vi "custom.vi"() -> ()   [LabVIEW 2009]
panel:
  out "Turning Turret":bool
  in  "Exit":bool
  in  "Abort\n Scan":bool
  out "Scanning":bool
  out "error out":errorcluster
  out "Status":string
  out "Emulating":bool
  out "Initialized":bool
  in  "Force\nInitialization":bool
  in  "Initialize":bool
  out "Current UniqueID":string
  in  "Mono ID":string(combo)
  in  "Switch \nTurret":bool
  out "Wavelength (nm)":dbl
  out "Grating Index":i32
  in  "Select Grating Blaze":string(combo)
  out "Current Blaze":string caption="Grating Blaze"
  out "Grating Density":dbl
  in  "Time Per Step":dbl=1.0 min=1.0 max=5000.0 step=1.0
  in  "Wavelength\n   Step Size":dbl=1.0 min=0.1 max=100.0
  in  "Ending\nWavelength":dbl=500.0 min=201.0 max=3000.0
  in  "Starting\nWavelength":dbl=450.0 min=18.0 max=2500.0
  in  "Target\nWavelength":dbl=450.0 min=18.0 max=3000.0
  in  "Increment":dbl=10.0 min=0.1 max=50.0
  out "Incrementing Down":bool
  out "Incrementing Up":bool
  out "Changing Wavelength":bool
  in  "Scan":bool
  in  "Increment Down":bool
  in  "Increment Up":bool
  in  "Change Wavelength":bool
  out "Drive Control Engaged":bool
  in  "Change \nGrating":bool
  in  "Enable\nDrive":bool
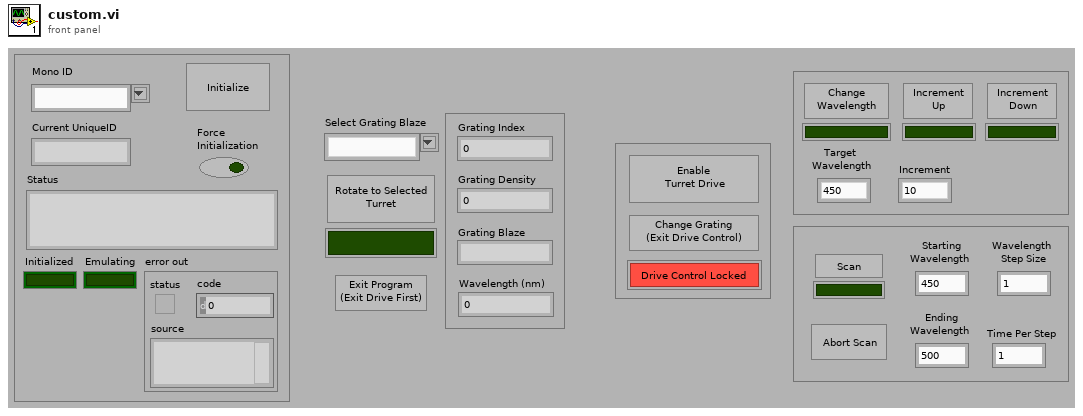
[diagram p1: front panel]
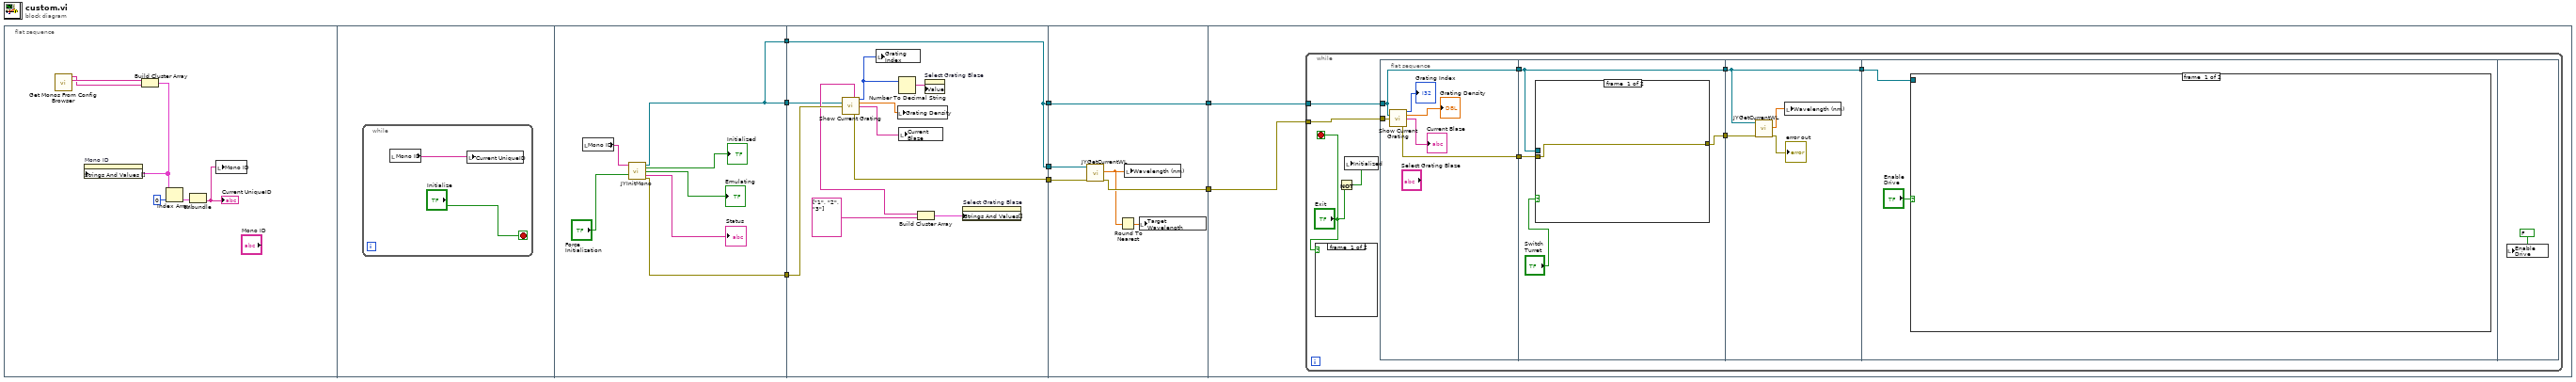
[diagram p0: block diagram]
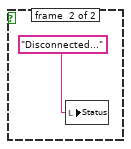
[diagram p2: hidden frame]
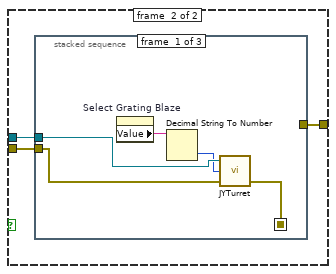
[diagram p3: hidden frame]
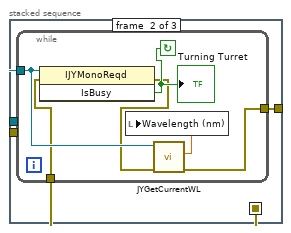
[diagram p4: hidden frame]
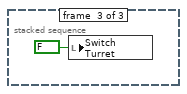
[diagram p5: hidden frame]
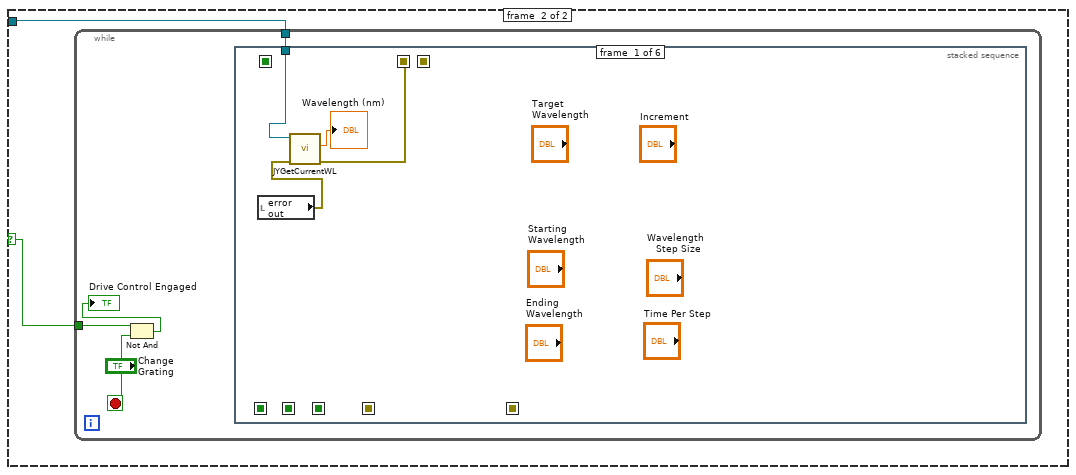
[diagram p6: hidden frame]
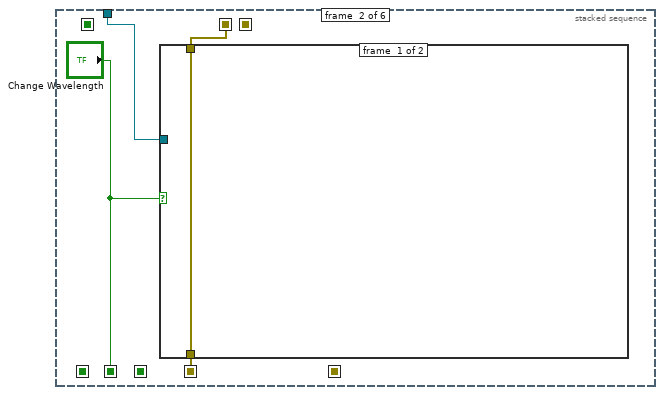
[diagram p7: hidden frame]
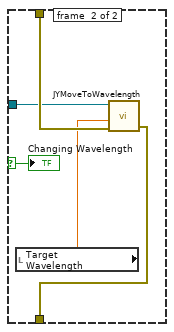
[diagram p8: hidden frame]
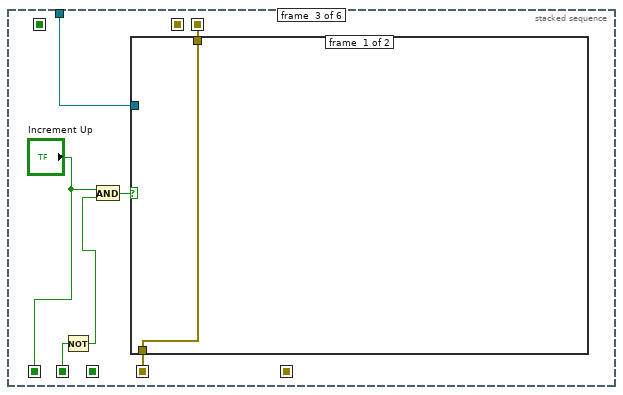
[diagram p9: hidden frame]
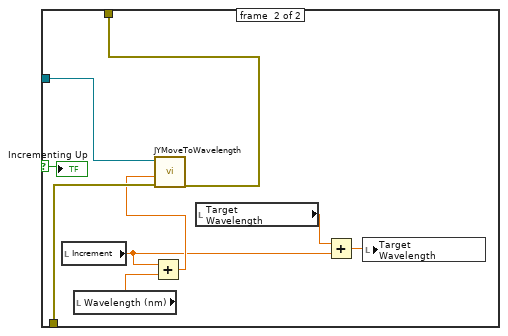
[diagram p10: hidden frame]
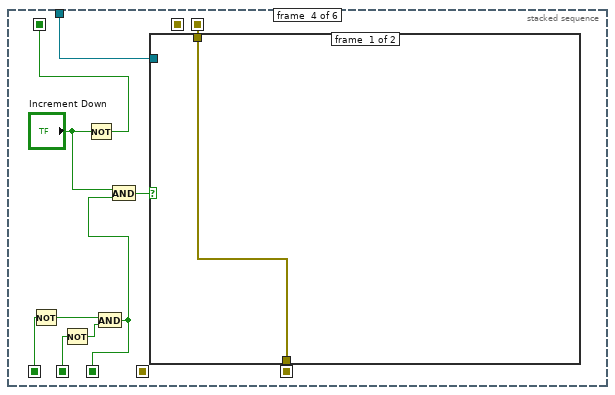
[diagram p11: hidden frame]
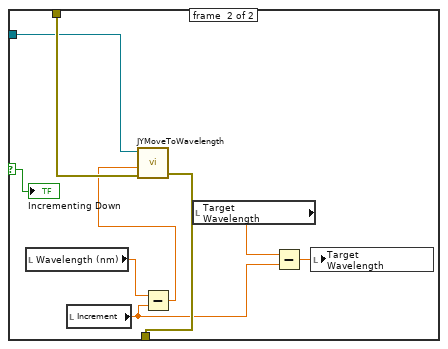
[diagram p12: hidden frame]
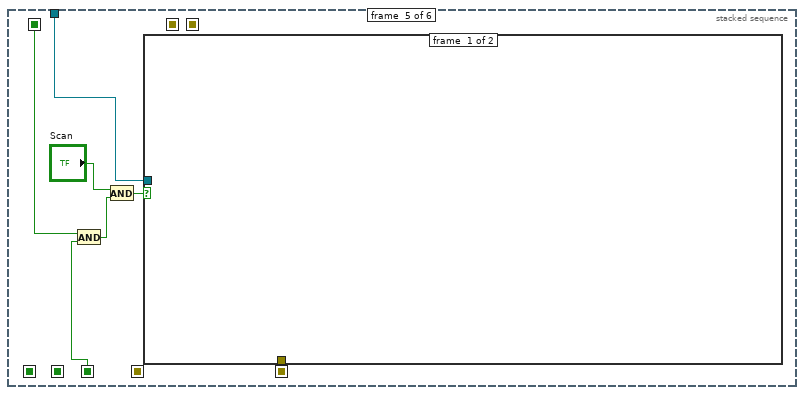
[diagram p13: hidden frame]
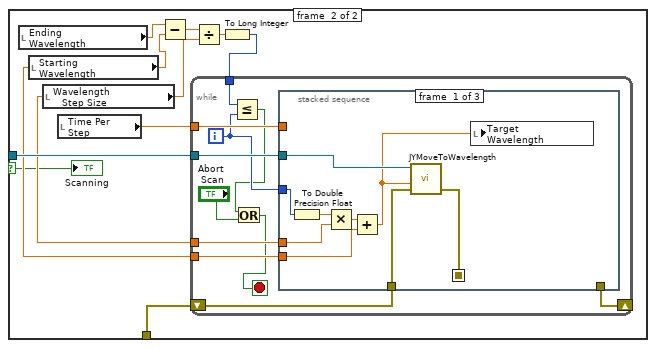
[diagram p14: hidden frame]
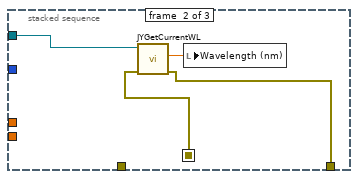
[diagram p15: hidden frame]
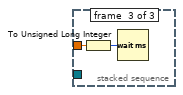
[diagram p16: hidden frame]
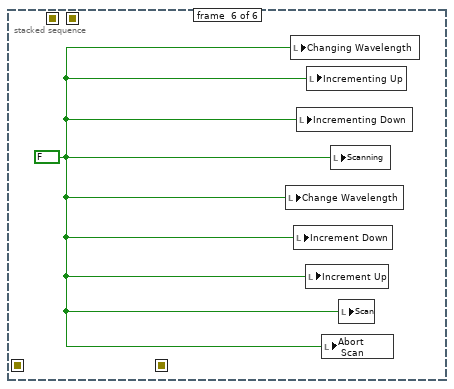
[diagram p17: hidden frame]
diagram:
  n1 = flat-sequence {
    tunnel: [w18] -> w8
    tunnel: [w17] -> w7
    tunnel: [w17] -> w2
    tunnel: w8 -> [w34]
    tunnel: w7 -> [w25]
    tunnel: [w32] -> w4
    tunnel: [w24] -> w6
    tunnel: w2 -> [w24]
    tunnel: [w24] -> w1
    tunnel: w6 -> [w40]
    tunnel: [w37] -> w5
    tunnel: w4 -> [w39]
    tunnel: [w38] -> w3
    tunnel: w1 -> [w37]
    tunnel: w5 -> [w41]
    tunnel: w3 -> [w42]
    frame #0 {
      n2 = call "Get Monos From Config Browser.vi"() -> ("UniqueIDs"=w13:string[], "Mono ID"=w14:string[])  [unwired: 3 in, 1 out]
      n3 = Build Cluster Array(w14, w13) -> (w11:cluster{"String":string, "String":string}[])
      n4 = property on="Mono ID" class="CmbBox"("Strings And Values []"=w11) -> ()  [unwired: 2 in, 2 out]
      n5 = Index Array(array=w11, index=0) -> (element=w12:cluster{"String":string, "String":string})
      n6 = Unbundle(w12) -> ("String"=w9:string)  [unwired: 1 out]
      "Current UniqueID" <- w9
      n7 = local write "Mono ID"(w9) -> ()
    }
    frame #1 {
      n8 = while {
        stop <- "Initialize" stop-if-true
        n9 = local read "Mono ID"() -> (w16:string)
        n10 = local write "Current UniqueID"(w16) -> ()
      }
    }
    frame #2 {
      n11 = local read "Mono ID"() -> (w22:string)
      n12 = call "JYInitMono.vi"("Unique ID"=w22, "Force Init"="Force\nInitialization") -> ("Mono RefNum out"=w17:refnum<k7>, "Initialized"=→"Initialized":bool, "Emulating"=→"Emulating":bool, "Status"=→"Status":string, "error out"=w18:errorcluster)  [unwired: 9 in]
    }
    frame #3 {
      n13 = call "Show Current Grating.vi"("Refnum in"=w25, "error in (no error)"=w34) -> ("Blazes"=w29:string[], "Grating Index"=w28:i32, "Current Grating"=w27:dbl, "Current Blaze"=w26:string, "error out"=w32:errorcluster)  [unwired: 5 in, 4 out]
      n14 = local write "Grating Index"(w28) -> ()
      n15 = local write "Grating Density"(w27) -> ()
      n16 = Number To Decimal String(number=w28) -> (decimal integer string=w31:string)  [unwired: 1 in]
      n17 = local write "Current Blaze"(w26) -> ()
      n18 = Build Cluster Array(w29, string[] ["1", "2", "3"]) -> (w30:cluster{"String":string, string}[])
      n19 = property on="Select Grating Blaze" class="CmbBox"("Value"=w31) -> ()  [unwired: 2 in, 2 out]
      n20 = property on="Select Grating Blaze" class="CmbBox"("Strings And Values[]"=w30) -> ()  [unwired: 2 in, 2 out]
    }
    frame #4 {
      n21 = call "JYGetCurrentWL.vi"("error in (no error)"=w39, "JYMONOLib.IJYMonoReqd"=w40) -> ("error out"=w38:errorcluster, "Current WL"=w36:dbl)  [unwired: 6 in, 2 out]
      n22 = Round To Nearest(number=w36) -> (nearest integer value=w35:dbl)
      n23 = local write "Wavelength (nm)"(w36) -> ()
      n24 = local write "Target\nWavelength"(w35) -> ()
    }
    frame #5 {
      n25 = while {
        tunnel: w41 -> [w51]
        tunnel: w42 -> [w50]
        stop <- "Exit" stop-if-true
        n26 = case shown="False" "Exit" {
          frame #0 {
          }
          frame #1 {
            n27 = local write "Status"("Disconnected...") -> ()
          }
        }
        n28 = Not(x="Exit") -> (.not. x?=w44:bool)
        n29 = local write "Initialized"(w44) -> ()
        n30 = flat-sequence {
          tunnel: w51 -> [w53]
          tunnel: w50 -> [w55]
          tunnel: [w54] -> w49
          tunnel: [w53] -> w47
          tunnel: w49 -> [w62]
          tunnel: [w60] -> w48
          tunnel: w47 -> [w61]
          tunnel: [w61] -> w46
          tunnel: w48 -> [w85]
          tunnel: w46 -> [w84]
          tunnel: [w84] -> w45
          tunnel: w45 -> [w87]
          frame #0 {
            n31 = call "Show Current Grating.vi"("Refnum in"=w53, "error in (no error)"=w55) -> ("Grating Index"=→"Grating Index":i32, "Current Grating"=→"Grating Density":dbl, "Current Blaze"=→"Current Blaze":string, "error out"=w54:errorcluster)  [unwired: 5 in, 5 out]
          }
          frame #1 {
            n32 = case shown="True" "Switch \nTurret" {
              tunnel: w62 -> [w63 w66]
              tunnel: w61 -> [_ w65]
              tunnel: [w63 w64] -> w60
              frame #0 {
              }
              frame #1 {
                n33 = stacked-sequence {
                  seq-local: [w69 _ _] -> [_ w73 _]
                  tunnel: w66 -> [w71 _ _]
                  tunnel: w65 -> [w70 w74 _]
                  tunnel: [_ w72 _] -> w64
                  frame #0 {
                    n34 = property on="Select Grating Blaze" class="CmbBox"() -> ("Value"=w68:string)  [unwired: 2 in, 2 out]
                    n35 = Decimal String To Number(string=w68) -> (number=w67:i32)  [unwired: 2 in, 1 out]
                    n36 = call "JYTurret.vi"("error in (no error)"=w71, "Grating Index"=w67, "RefNum In"=w70) -> ("error out"=w69:errorcluster)  [unwired: 2 out]
                  }
                  frame #1 {
                    n37 = while {
                      tunnel: w74 -> [w80]
                      tunnel: w73 -> [w78]
                      tunnel: [w75] -> w72
                      stop <- w77 continue-if-true
                      n38 = invoke class="IJYMonoReqd" method="IsBusy"(reference=w80, error in=w78) -> (error out=w76:errorcluster, "IsBusy"=w77:bool)  [unwired: 1 in, 1 out]
                      "Turning Turret" <- w77
                      n39 = call "JYGetCurrentWL.vi"("error in (no error)"=w76, "JYMONOLib.IJYMonoReqd"=w80) -> ("error out"=w75:errorcluster, "Current WL"=w79:dbl)  [unwired: 6 in, 2 out]
                      n40 = local write "Wavelength (nm)"(w79) -> ()
                    }
                  }
                  frame #2 {
                    n41 = local write "Switch \nTurret"(FALSE ("Switch \nTurret")) -> ()
                  }
                }
              }
            }
          }
          frame #2 {
            n42 = call "JYGetCurrentWL.vi"("error in (no error)"=w85, "JYMONOLib.IJYMonoReqd"=w84) -> ("error out"=→"error out":errorcluster, "Current WL"=w82:dbl)  [unwired: 6 in, 2 out]
            n43 = local write "Wavelength (nm)"(w82) -> ()
          }
          frame #3 {
            n44 = case shown="False" "Enable\nDrive" {
              selector: "Enable\nDrive" -> [_ w89]
              tunnel: w87 -> [_ w88]
              frame #0 {
              }
              frame #1 {
                n45 = while {
                  tunnel: w89 -> [w91]
                  tunnel: w88 -> [w90]
                  stop <- "Change \nGrating" stop-if-true
                  n46 = Not And(1:"Change \nGrating", 2:w91) -> (0:→"Drive Control Engaged":bool)
                  n47 = stacked-sequence {
                    seq-local: [_ "Change Wavelength" _ _ _ _] -> [_ _ w114 w135 _ _]
                    seq-local: [_ _ "Increment Up" _ _ _] -> [_ _ _ w134 _ _]
                    seq-local: [_ _ _ w129 _ _] -> [_ _ _ _ w152 _]
                    seq-local: [_ _ _ w128 _ _] -> [_ _ _ _ w151 _]
                    seq-local: [w95 _ _ _ _ _] -> [_ w100 _ _ _ _]
                    seq-local: [_ w98 _ _ _ _] -> [_ _ w110 _ _ _]
                    seq-local: [_ _ w108 _ _ _] -> [_ _ _ w127 _ _]
                    seq-local: [_ _ _ w125 _ _] -> [_ _ _ _ w147 _]
                    tunnel: w90 -> [w94 w99 w109 w126 w146 _]
                    frame #0 {
                      n48 = local read "error out"() -> (w97:errorcluster)
                      n49 = call "JYGetCurrentWL.vi"("error in (no error)"=w97, "JYMONOLib.IJYMonoReqd"=w94) -> ("error out"=w95:errorcluster, "Current WL"=→"Wavelength (nm)":dbl)  [unwired: 6 in, 2 out]
                    }
                    frame #1 {
                      n50 = case shown="True" "Change Wavelength" {
                        selector: "Change Wavelength" -> [_ w103]
                        tunnel: w100 -> [w102 w107]
                        tunnel: w99 -> [_ w106]
                        tunnel: [w102 w105] -> w98
                        frame #0 {
                        }
                        frame #1 {
                          n51 = local read "Target\nWavelength"() -> (w104:dbl)
                          n52 = call "JYMoveToWavelength.vi"("error in (no error)"=w107, "Target WL"=w104, "RefNum In"=w106) -> ("error out"=w105:errorcluster)  [unwired: 1 in, 2 out]
                          "Changing Wavelength" <- w103
                        }
                      }
                    }
                    frame #2 {
                      n53 = Not(x=w114) -> (.not. x?=w111:bool)
                      n54 = And(x="Increment Up", y=w111) -> (x .and. y?=w113:bool)
                      n55 = case shown="True" w113 {
                        selector: w113 -> [_ w116]
                        tunnel: w110 -> [w115 w124]
                        tunnel: w109 -> [_ w122]
                        tunnel: [w115 w121] -> w108
                        frame #0 {
                        }
                        frame #1 {
                          n56 = local read "Increment"() -> (w119:dbl)
                          n57 = local read "Wavelength (nm)"() -> (w120:dbl)
                          n58 = Add(x=w119, y=w120) -> (x+y=w123:dbl)
                          n59 = call "JYMoveToWavelength.vi"("error in (no error)"=w124, "Target WL"=w123, "RefNum In"=w122) -> ("error out"=w121:errorcluster)  [unwired: 1 in, 2 out]
                          n60 = local read "Target\nWavelength"() -> (w118:dbl)
                          n61 = Add(x=w118, y=w119) -> (x+y=w117:dbl)
                          n62 = local write "Target\nWavelength"(w117) -> ()
                          "Incrementing Up" <- w116
                        }
                      }
                    }
                    frame #3 {
                      n63 = Not(x=w134) -> (.not. x?=w132:bool)
                      n64 = Not(x=w135) -> (.not. x?=w133:bool)
                      n65 = Not(x="Increment Down") -> (.not. x?=w129:bool)
                      n66 = And(x=w132, y=w133) -> (x .and. y?=w128:bool)
                      n67 = And(x="Increment Down", y=w128) -> (x .and. y?=w131:bool)
                      n68 = case shown="True" w131 {
                        selector: w131 -> [_ w137]
                        tunnel: w127 -> [w136 w145]
                        tunnel: w126 -> [_ w143]
                        tunnel: [w136 w142] -> w125
                        frame #0 {
                        }
                        frame #1 {
                          n69 = local read "Wavelength (nm)"() -> (w141:dbl)
                          n70 = local read "Increment"() -> (w139:dbl)
                          n71 = Subtract(x=w141, y=w139) -> (x-y=w144:dbl)
                          n72 = call "JYMoveToWavelength.vi"("error in (no error)"=w145, "Target WL"=w144, "RefNum In"=w143) -> ("error out"=w142:errorcluster)  [unwired: 1 in, 2 out]
                          n73 = local read "Target\nWavelength"() -> (w140:dbl)
                          n74 = Subtract(x=w140, y=w139) -> (x-y=w138:dbl)
                          n75 = local write "Target\nWavelength"(w138) -> ()
                          "Incrementing Down" <- w137
                        }
                      }
                    }
                    frame #4 {
                      n76 = And(x=w152, y=w151) -> (x .and. y?=w149:bool)
                      n77 = And(x="Scan", y=w149) -> (x .and. y?=w150:bool)
                      n78 = case shown="True" w150 {
                        selector: w150 -> [_ w153]
                        tunnel: w147 -> [_ w158]
                        tunnel: w146 -> [_ w157]
                        frame #0 {
                        }
                        frame #1 {
                          n79 = local read "Ending\nWavelength"() -> (w160:dbl)
                          n80 = local read "Starting\nWavelength"() -> (w155:dbl)
                          n81 = local read "Wavelength\n   Step Size"() -> (w156:dbl)
                          n82 = local read "Time Per Step"() -> (w159:dbl)
                          n83 = Subtract(x=w160, y=w155) -> (x-y=w162:dbl)
                          n84 = Divide(x=w162, y=w156) -> (x/y=w161:dbl)
                          n85 = To Long Integer(number=w161) -> (32bit integer=w154:i32)
                          n86 = while {
                            tunnel: w155 -> [w169]
                            tunnel: w159 -> [w173]
                            shift-right: [w168] -> _
                            shift-left: w158 -> [w172]
                            tunnel: w157 -> [w171]
                            tunnel: w156 -> [w170]
                            tunnel: w154 -> [w164]
                            i -> [w167]
                            stop <- w165 stop-if-true
                            n87 = Less Or Equal?(x=w164, y=w167) -> (x <= y?=w166:bool)
                            n88 = Or(x=w166, y="Abort\n Scan") -> (x .or. y?=w165:bool)
                            n89 = stacked-sequence {
                              seq-local: [w175 _ _] -> [_ w184 _]
                              tunnel: w173 -> [_ _ w187]
                              tunnel: w172 -> [w182 _ _]
                              tunnel: w171 -> [w181 w185 _]
                              tunnel: w170 -> [w180 _ _]
                              tunnel: w167 -> [w179 _ _]
                              tunnel: w169 -> [w176 _ _]
                              tunnel: [_ w183 _] -> w168
                              frame #0 {
                                n90 = To Double Precision Float(number=w179) -> (double precision float=w178:dbl)
                                n91 = Multiply(x=w178, y=w180) -> (x*y=w177:dbl)
                                n92 = Add(x=w177, y=w176) -> (x+y=w174:dbl)
                                n93 = call "JYMoveToWavelength.vi"("error in (no error)"=w182, "Target WL"=w174, "RefNum In"=w181) -> ("error out"=w175:errorcluster)  [unwired: 1 in, 2 out]
                                n94 = local write "Target\nWavelength"(w174) -> ()
                              }
                              frame #1 {
                                n95 = call "JYGetCurrentWL.vi"("error in (no error)"=w184, "JYMONOLib.IJYMonoReqd"=w185) -> ("error out"=w183:errorcluster, "Current WL"=w186:dbl)  [unwired: 6 in, 2 out]
                                n96 = local write "Wavelength (nm)"(w186) -> ()
                              }
                              frame #2 {
                                n97 = To Unsigned Long Integer(number=w187) -> (unsigned 32bit integer=w188:u32)
                                n98 = Wait (ms)(milliseconds to wait=w188) -> ()  [unwired: 1 out]
                              }
                            }
                          }
                          "Scanning" <- w153
                        }
                      }
                    }
                    frame #5 {
                      w189 = FALSE
                      n99 = local write "Change Wavelength"(w189) -> ()
                      n100 = local write "Changing Wavelength"(w189) -> ()
                      n101 = local write "Increment Down"(w189) -> ()
                      n102 = local write "Incrementing Down"(w189) -> ()
                      n103 = local write "Increment Up"(w189) -> ()
                      n104 = local write "Incrementing Up"(w189) -> ()
                      n105 = local write "Abort\n Scan"(w189) -> ()
                      n106 = local write "Scanning"(w189) -> ()
                      n107 = local write "Scan"(w189) -> ()
                    }
                  }
                }
              }
            }
          }
          frame #4 {
            n108 = local write "Enable\nDrive"(FALSE) -> ()
          }
        }
      }
    }
  }
